vi "Terminal-PressureSystem-LoadingUnit-Getter.vi"(8 "error in (no error)":errorcluster caption="错误输入（无错误）", 11 "read operation timeout (ms)":i32=5000 caption="读操作超时（5000毫秒）") -> (0 "error out":errorcluster caption="错误输出", 2 "时间标识":timestamp, 3 "液压子系统比例加载单元":T1)   [LabVIEW 2014]
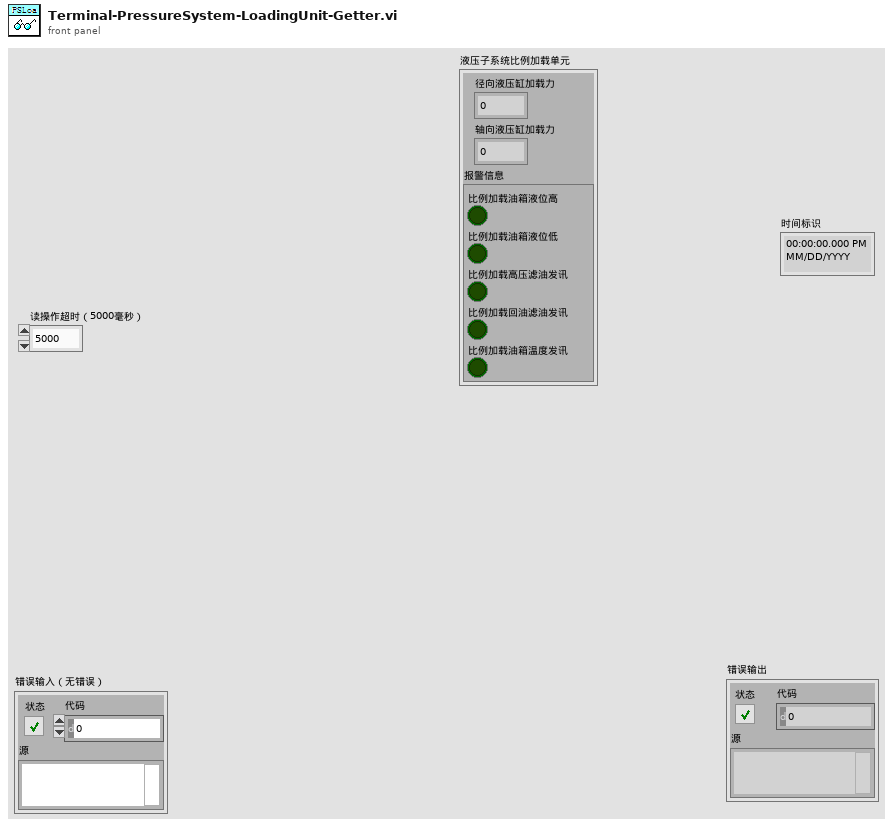
[diagram p1: front panel]
types:
  T1 = cluster{"径向液压缸加载力":u16, "轴向液压缸加载力":u16, "报警信息":cluster{"比例加载油箱液位高":bool, "比例加载油箱液位低":bool, "比例加载高压滤油发讯":bool, "比例加载回油滤油发讯":bool, "比例加载油箱温度发讯":bool}}
  T2 = cluster{"比例加载油箱液位高":bool, "比例加载油箱液位低":bool, "比例加载高压滤油发讯":bool, "比例加载回油滤油发讯":bool, "比例加载油箱温度发讯":bool}
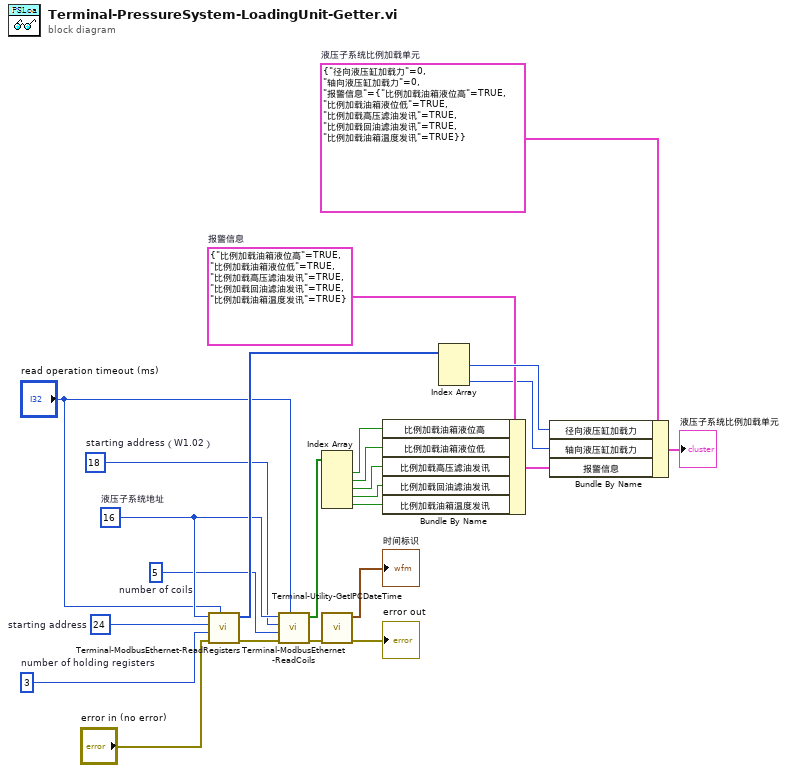
[diagram p0: block diagram]
diagram:
  w10 = T2 {"比例加载油箱液位高"=TRUE, "比例加载油箱液位低"=TRUE, "比例加载高压滤油发讯"=TRUE, "比例加载回油滤油发讯"=TRUE, "比例加载油箱温度发讯"=TRUE}  # 报警信息
  w13 = u16 5  # number of coils
  w14 = u16 18  # starting address（W1.02）
  w22 = T1 {"径向液压缸加载力"=0, "轴向液压缸加载力"=0, "报警信息"={"比例加载油箱液位高"=TRUE, "比例加载油箱液位低"=TRUE, "比例加载高压滤油发讯"=TRUE, "比例加载回油滤油发讯"=TRUE, "比例加载油箱温度发讯"=TRUE}}  # 液压子系统比例加载单元
  w3 = u16 3  # number of holding registers
  w24 = u16 24  # starting address
  w15 = u8 16  # 液压子系统地址
  n1 = call "Terminal-ModbusEthernet-ReadRegisters.vi"("read operation timeout (ms)"="read operation timeout (ms)", "error in"="error in (no error)", "number of holding registers"=w3, "starting address"=w24, "unit ID"=w15) -> ("error out"=w2:errorcluster, "register values"=w18:u16[])  [unwired: 5 in]
  n2 = call "Terminal-ModbusEthernet-ReadCoils.vi"("read operation timeout (ms)"="read operation timeout (ms)", "error in"=w2, "number of coils"=w13, "starting address"=w14, "unit ID"=w15) -> ("error out"=w16:errorcluster, "coil values"=w12:bool[])  [unwired: 5 in]
  n3 = Index Array(array=w12) -> (element #1=w8:bool, element #2=w7:bool, element #3=w6:bool, element #4=w5:bool, element #5=w4:bool)  [unwired: 5 in]
  n4 = call "Terminal-Utility-GetIPCDateTime.vi"("error in (no error)"=w16) -> ("error out"=→"error out":errorcluster, "时间标识"=→"时间标识":timestamp)  [unwired: 9 in]
  n5 = Bundle By Name(cluster=w10, "比例加载油箱液位高"=w8, "比例加载油箱液位低"=w7, "比例加载高压滤油发讯"=w6, "比例加载回油滤油发讯"=w5, "比例加载油箱温度发讯"=w4) -> (w9:T2)
  n6 = Index Array(array=w18) -> (element #1=w21:u16, element #3=w1:u16)  [unwired: 3 in, 1 out]
  n7 = Bundle By Name(cluster=w22, "径向液压缸加载力"=w21, "轴向液压缸加载力"=w1, "报警信息"=w9) -> (→"液压子系统比例加载单元":T1)
